vi "Save Settings to XML.vi"(8 "error in (no error)":errorcluster, 11 "Settings":T1={"Acquisition Settings"={"AI"={"task name"="", "task_ref"="", "physical channels"="Dev1/ai0:7", "channels config"={"input terminal configuration"=0, "minimum value"=-5.0, "maximum value"=5.0}, "rate"=1000.0}, "conversions"={"ai0"={"a"=0.0, "b"=0.0}, "ai1"={"a"=0.0, "b"=0.0}, "ai2"={"a"=0.0, "b"=0.0}, "ai3"={"a"=0.0, "b"=0.0}, "ai4"={"a"=0.0, "b"=0.0}}, "compteur 0"={"task name"="CTR", "task_ref"="", "ctr"="Dev1/ctr0:3", "coeff"=4000.0}, "compteur 1"={"task name"="CTR1", "task_ref"="", "ctr"="Dev1/ctr1", "coeff"=4000.0}, "compteur 2"={"task name"="CTR2", "task_ref"="", "ctr"="Dev1/ctr2", "coeff"=4000.0}, "compteur 3"={"task name"="CTR3", "task_ref"="", "ctr"="Dev1/ctr3", "coeff"=4000.0}}, "Logging Configuration"={"Log File Base Path"=path "", "L1"={"ref"=refnum, "actif?"=FALSE, "Fsave"=0.0}, "L2"={"ref"=refnum, "actif?"=FALSE, "Fsave"=0.0}, "L3"={"ref"=refnum, "actif?"=FALSE, "Fsave"=0.0}, "L4"={"ref"=refnum, "actif?"=FALSE, "Fsave"=0.0}}, "Generation Settings"={"AO"={"task name"="AO", "task_ref"="", "physical channels"="Dev1/ao0"}, "PID"={"P"=0.0, "I"=0.0, "D"=0.0}, "conversions"={"ao0"={"a"=0.0, "b"=0.0}}, "setpoint"=0.0}, "Digital Control Configuration"={"DO"={"task name"="DO", "task_ref"="", "lines"="Dev1/port0/line2:3, Dev1/port0/line5"}}} {"Acquisition Settings"."compteur 3"."coeff" format="%0.2f"; "Acquisition Settings"."compteur 2"."coeff" format="%0.2f"; "Acquisition Settings"."compteur 1"."coeff" format="%0.2f"; "Acquisition Settings"."compteur 0"."coeff" format="%0.2f"; "Acquisition Settings"."AI"."rate" format="%0.2f"; "Acquisition Settings"."AI"."channels config"."input terminal configuration" items=["Default"=-1, "RSE"=10083, "NRSE"=10078, "Differential"=10106, "Pseudodifferential"=12529]}) -> (0 "error out":errorcluster)   [LabVIEW 2014, in "PLS Settings.lvlib"]
doc: "Saves the \"User Specified\" configuration data to an XML file. This is used to remember the users settings between executions."
uses:
  PLS Settings.lvlib
  Settings.ctl
  Acquisition/Hardware Configuration.ctl
  conversion.ctl
  Logging/Logging Configuration.ctl
  Generation/Hardware Configuration.ctl
  Digital Control/Hardware Configuration.ctl
  <vilib>/Utility/xml.llb/Write to XML File(string).vi
  Acquisition/PLS Acquisition.lvlib
  Logging/PLS Logging.lvlib
  Generation/PLS Generation.lvlib
  Digital Control/PLS Digital Control.lvlib
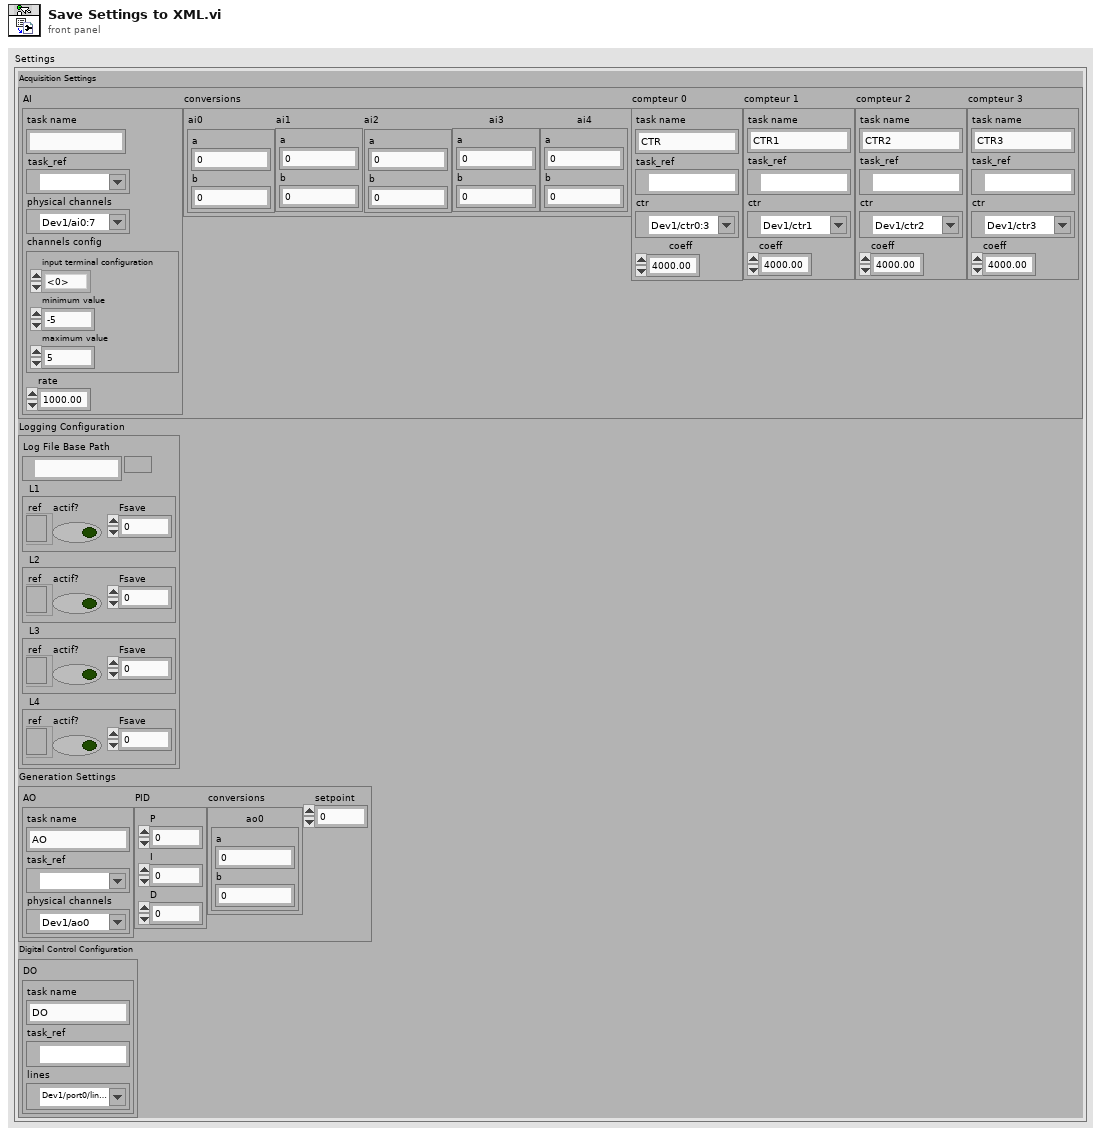
[diagram p1: front panel]
types:
  T1 = typedef "PLS Settings.lvlib/Settings.ctl" = cluster{"Acquisition Settings":T2, "Logging Configuration":T4, "Generation Settings":T5, "Digital Control Configuration":T6}
  T2 = typedef "PLS Acquisition.lvlib/Hardware Configuration.ctl" = cluster{"AI":cluster{"task name":string, "task_ref":refnum<k21>, "physical channels":tag, "channels config":cluster{"input terminal configuration":i32, "minimum value":dbl, "maximum value":dbl}, "rate":dbl}, "conversions":cluster{"ai0":T3, "ai1":T3, "ai2":T3, "ai3":T3, "ai4":T3}, "compteur 0":cluster{"task name":string, "task_ref":refnum<k21>, "ctr":tag, "coeff":dbl}, "compteur 1":cluster{"task name":string, "task_ref":refnum<k21>, "ctr":tag, "coeff":dbl}, "compteur 2":cluster{"task name":string, "task_ref":refnum<k21>, "ctr":tag, "coeff":dbl}, "compteur 3":cluster{"task name":string, "task_ref":refnum<k21>, "ctr":tag, "coeff":dbl}}
  T3 = typedef "PLS Settings.lvlib/conversion.ctl" = cluster{"a":dbl, "b":dbl}
  T4 = typedef "PLS Logging.lvlib/Logging Configuration.ctl" = cluster{"Log File Base Path":path, "L1":cluster{"ref":refnum<file>, "actif?":bool, "Fsave":dbl}, "L2":cluster{"ref":refnum<file>, "actif?":bool, "Fsave":dbl}, "L3":cluster{"ref":refnum<file>, "actif?":bool, "Fsave":dbl}, "L4":cluster{"ref":refnum<file>, "actif?":bool, "Fsave":dbl}}
  T5 = typedef "PLS Generation.lvlib/Hardware Configuration.ctl" = cluster{"AO":cluster{"task name":string, "task_ref":refnum<k21>, "physical channels":tag}, "PID":cluster{"P":dbl, "I":dbl, "D":dbl}, "conversions":cluster{"ao0":T3}, "setpoint":dbl}
  T6 = typedef "PLS Digital Control.lvlib/Hardware Configuration.ctl" = cluster{"DO":cluster{"task name":string, "task_ref":refnum<k21>, "lines":tag}}
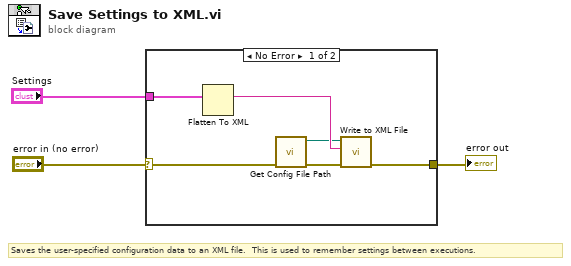
[diagram p0: block diagram]
diagram:
  # "Saves the user-specified configuration data to an XML file.  This is used to remember settings between executions."
  n1 = case shown="No Error" "error in (no error)" {
    selector: "error in (no error)" -> [w5 w10]
    tunnel: [w7 w10] -> w2
    tunnel: "Settings" -> [w9 _]
    frame No Error {
      n2 = Flatten To XML(anything=w9) -> (xml string=w8:string)
      n3 = call "Get Config File Path.vi"("error in (no error)"=w5) -> ("error out"=w4:errorcluster, "XML File Path"=w6:path)  [unwired: 9 in]
      n4 = call-poly <vilib>:"Write to XML File.vi"("error in (no error)"=w4, "XML Input"=w8, "XML File Path"=w6) -> ("error out"=w7:errorcluster)  [unwired: 6 in, 2 out]
    }
    frame Error {
    }
  }
  "error out" <- w2
